vi "SGSA_Freq_Sweep_Only.vi"() -> ()   [LabVIEW 2023, in "SG_SA.lvlib"]
uses:
  SG_SA.lvlib
  lib/Keysight/Keysight.lvlib
panel:
  in  "IF(MHz)":i32=100
  in  "Average Times":i32=5
  in  "Waiting Time(ms)":u32=1000
  in  "Stop Freq.(MHz)":i32=28000
  in  "Start Freq.(MHz)":i32=27000
  in  "Steps(MHz)":i32=100
  in  "FileNote":string
  in  "SG":refnum<visa-resource-name>="TCPIP0::192.168.100.201::inst0::INSTR"
  in  "SA":refnum<visa-resource-name>="TCPIP0::192.168.100.202::hislip0::INSTR"
  out "SA Freq(MHz)":i32
  out "SG Freq(MHz)":i32
  out "Spectrum Data":cluster{"X":dbl, "Y":dbl}[](graph)
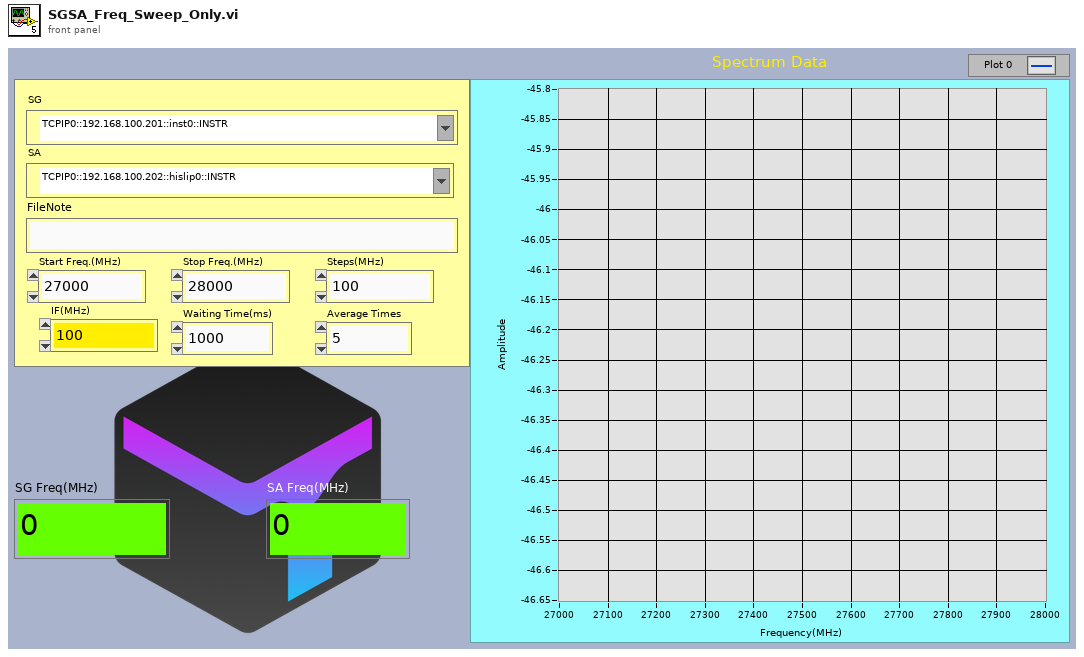
[diagram p1: front panel]
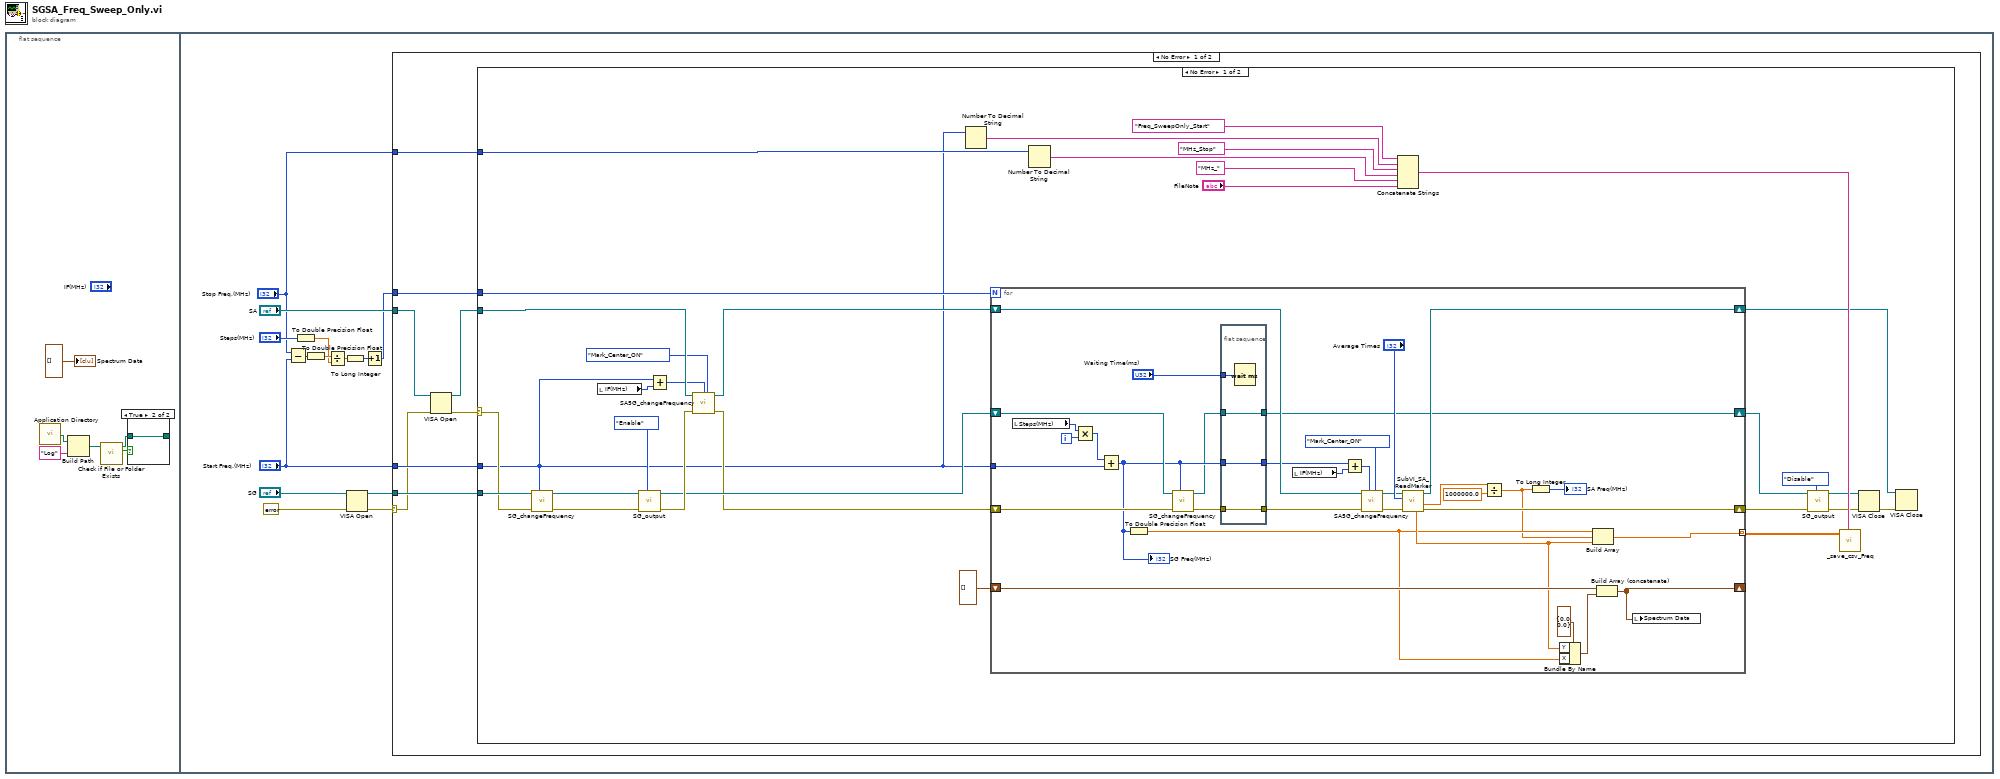
[diagram p0: block diagram]
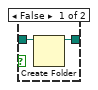
[diagram p2: hidden frame]
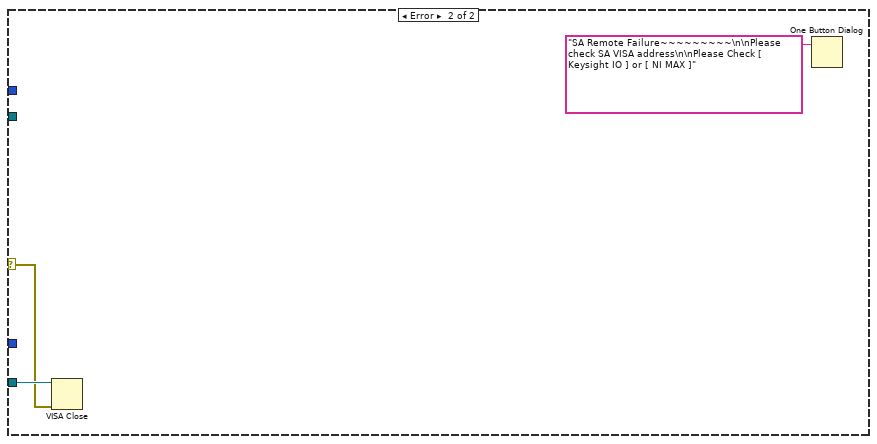
[diagram p3: hidden frame]
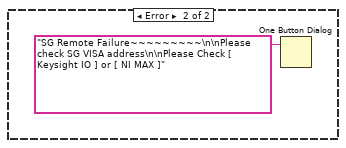
[diagram p4: hidden frame]
diagram:
  n1 = flat-sequence {
    frame #0 {
      n2 = call <vilib>:"Application Directory.vi"() -> ("Application Directory"=w5:path)
      n3 = Build Path(base path=w5, name or relative path="Log") -> (appended path=w2:path)
      n4 = call <vilib>:"Check if File or Folder Exists.vi"("path"=w2) -> ("file or folder exists?"=w4:bool, "dup path"=w3:path)  [unwired: 8 in, 1 out]
      n5 = case shown="True" w4 {
        tunnel: w3 -> [w8 w9]
        tunnel: [w7 w9] -> _
        frame False {
          n6 = Create Folder(path (use dialog)=w8) -> (created path=w7:path)  [unwired: 2 in, 2 out]
        }
        frame True {
        }
      }
      "Spectrum Data" <- cluster{"X":dbl, "Y":dbl}[] [] ("XY Graph")
    }
    frame #1 {
      n7 = Subtract(x="Stop Freq.(MHz)", y="Start Freq.(MHz)") -> (x-y=w16:i32)
      n8 = To Double Precision Float(number="Steps(MHz)") -> (double precision float=w11:dbl)
      n9 = To Double Precision Float(number=w16) -> (double precision float=w12:dbl)
      n10 = Divide(x=w12, y=w11) -> (x/y=w14:dbl)
      n11 = To Long Integer(number=w14) -> (32bit integer=w13:i32)
      n12 = VISA Open(error in (no error)=errorcluster {"status"=FALSE, "code"=0, "source"=""}, VISA resource name="SG") -> (VISA resource name=w18:refnum<visa-resource-name>, error out=w17:errorcluster)  [unwired: 3 in]
      n13 = Increment(x=w13) -> (x+1=w21:i32)
      n14 = case shown="No Error" w17 {
        selector: w17 -> [w28 _]
        tunnel: "SA" -> [w26 _]
        tunnel: "Start Freq.(MHz)" -> [w31 _]
        tunnel: w21 -> [w30 _]
        tunnel: w18 -> [w29 _]
        tunnel: "Stop Freq.(MHz)" -> [w24 _]
        frame No Error {
          n15 = VISA Open(error in (no error)=w28, VISA resource name=w26) -> (VISA resource name=w25:refnum<visa-resource-name>, error out=w27:errorcluster)  [unwired: 3 in]
          n16 = case shown="No Error" w27 {
            selector: w27 -> [w60 w101]
            tunnel: w25 -> [w63 _]
            tunnel: w31 -> [w34 _]
            tunnel: w30 -> [w62 _]
            tunnel: w29 -> [w61 w102]
            tunnel: w24 -> [w37 _]
            frame No Error {
              n17 = call "SG_changeFrequency.vi"("MHz"=w34, "error in"=w60, "VISA in"=w61) -> ("error out"=w42:errorcluster, "VISA out"=w40:refnum<visa-resource-name>)  [unwired: 6 in, 1 out]
              n18 = local read "IF(MHz)"() -> (w32:i32)
              n19 = call "SG_output.vi"("Func."=enum16{"Disable", "Enable"}."Enable", "error in"=w42, "VISA in"=w40) -> ("error out"=w41:errorcluster, "VISA out"=w39:refnum<visa-resource-name>)  [unwired: 7 in]
              n20 = Add(x=w34, y=w32) -> (x+y=w33:i32)
              n21 = call "SA5G_changeFrequency.vi"("Enum"=enum16{"Mark_Center_OFF", "Mark_Center_ON"}."Mark_Center_ON", "MHz"=w33, "error in"=w41, "VISA in"=w63) -> ("error out"=w38:errorcluster, "VISA out"=w54:refnum<visa-resource-name>)  [unwired: 5 in, 1 out]
              n22 = Number To Decimal String(number=w34) -> (decimal integer string=w51:string)  [unwired: 1 in]
              n23 = for {
                N: w62 -> [_]
                shift-right: [w96] -> w49
                shift-left: w38 -> [w88]
                shift-right: [w71] -> w48
                shift-left: w39 -> [w86]
                tunnel: [w94] -> w58 mode=indexing
                shift-right: [w93] -> w55
                shift-left: w54 -> [w75]
                shift-right: [w89] -> _
                shift-left: cluster{"X":dbl, "Y":dbl}[] [] ("XY Graph") -> [w91]
                tunnel: w34 -> [w81]
                i -> [w83]
                n24 = local read "Steps(MHz)"() -> (w84:i32)
                n25 = Multiply(x=w84, y=w83) -> (x*y=w82:i32)
                n26 = Add(x=w82, y=w81) -> (x+y=w73:i32)
                "SG Freq(MHz)" <- w73
                n27 = To Double Precision Float(number=w73) -> (double precision float=w69:dbl)
                n28 = call "SG_changeFrequency.vi"("MHz"=w73, "error in"=w88, "VISA in"=w86) -> ("error out"=w87:errorcluster, "VISA out"=w72:refnum<visa-resource-name>)  [unwired: 6 in, 1 out]
                n29 = flat-sequence {
                  tunnel: w87 -> [w100]
                  tunnel: [w100] -> w76
                  tunnel: "Waiting Time(ms)" -> [w99]
                  tunnel: w73 -> [w98]
                  tunnel: [w98] -> w64
                  tunnel: w72 -> [w97]
                  tunnel: [w97] -> w71
                  frame #0 {
                    n30 = Wait (ms)(milliseconds to wait=w99) -> ()  [unwired: 1 out]
                  }
                }
                n31 = local read "IF(MHz)"() -> (w66:i32)
                n32 = Add(x=w64, y=w66) -> (x+y=w65:i32)
                n33 = call "SA5G_changeFrequency.vi"("Enum"=enum16{"Mark_Center_OFF", "Mark_Center_ON"}."Mark_Center_ON", "MHz"=w65, "error in"=w76, "VISA in"=w75) -> ("error out"=w77:errorcluster, "VISA out"=w74:refnum<visa-resource-name>)  [unwired: 5 in, 1 out]
                n34 = call "SubVI_SA_ReadMarker.vi"("error in (no error)"=w77, "AvgTimes"="Average Times", "VISA resource name"=w74) -> ("error out"=w96:errorcluster, "Marker Freq."=w80:dbl, "VISA resource name out"=w93:refnum<visa-resource-name>, "Marker Power"=w78:dbl)  [unwired: 5 in]
                n35 = Divide(x=w80, y=1000000.0) -> (x/y=w68:dbl)
                n36 = To Long Integer(number=w68) -> (32bit integer=→"SA Freq(MHz)":i32)
                n37 = Bundle By Name(cluster=cluster{"X":dbl, "Y":dbl} {"X"=0.0, "Y"=0.0} ("element"), "Y"=w78, "X"=w69) -> (w90:cluster{"X":dbl, "Y":dbl})
                n38 = Build Array(w69, w68, w78) -> (w94:dbl[])
                n39 = Build Array (concatenate)(w91, w90) -> (w89:cluster{"X":dbl, "Y":dbl}[])
                n40 = local write "Spectrum Data"(w89) -> ()
              }
              n41 = Number To Decimal String(number=w37) -> (decimal integer string=w36:string)  [unwired: 1 in]
              n42 = Concatenate Strings("Freq_SweepOnly_Start" ("delimiter (\\t)"), w51, "MHz_Stop", w36, "MHz_", "FileNote") -> (w59:string)
              n43 = call "SG_output.vi"("Func."=enum16{"Disable", "Enable"}."Disable", "error in"=w49, "VISA in"=w48) -> ("error out"=w46:errorcluster, "VISA out"=w47:refnum<visa-resource-name>)  [unwired: 7 in]
              n44 = call "_save_csv_Freq.vi"("delimiter (\\t)"=w59, "Data"=w58) -> ()  [unwired: 9 in, 1 out]
              n45 = VISA Close(VISA resource name=w47, error in (no error)=w46) -> (error out=w56:errorcluster)
              n46 = VISA Close(VISA resource name=w55, error in (no error)=w56) -> ()  [unwired: 1 out]
            }
            frame Error {
              n47 = VISA Close(VISA resource name=w102, error in (no error)=w101) -> ()  [unwired: 1 out]
              n48 = One Button Dialog(message="SA Remote Failure~~~~~~~~~\n\nPlease check SA VISA address\n\nPlease Check [ Keysight IO ] or [ NI MAX ]") -> ()  [unwired: 1 in, 1 out]
            }
          }
        }
        frame Error {
          n49 = One Button Dialog(message="SG Remote Failure~~~~~~~~~\n\nPlease check SG VISA address\n\nPlease Check [ Keysight IO ] or [ NI MAX ]") -> ()  [unwired: 1 in, 1 out]
        }
      }
    }
  }
